vi "Process GD Infos.vi"(5 "include Timestamp":bool, 7 "show Status even if no Error":bool, 8 "Sprachliste":string[][](array[string]), 9 "GD Info-Cluster in":T1, 10 "Array (Eingang)":string[](array[string]), 11 "Error occured (Eingang)":bool) -> (1 "GD Infos":string, 2 "Array (Ausgang)":string[](array[string]), 3 "Error occured (Ausgang)":bool)   [LabVIEW 2020, in "Linearisierung v2.lvlib" / "SpanEinstellungen.lvlib"]
uses:
  SpanEinstellungen.lvlib
  GD Info Cluster.ctl
  LIN ErrorCluster.ctl
  Sprachverwaltung/Sprachverwaltung.lvlib
  Linearisierung v2.lvlib
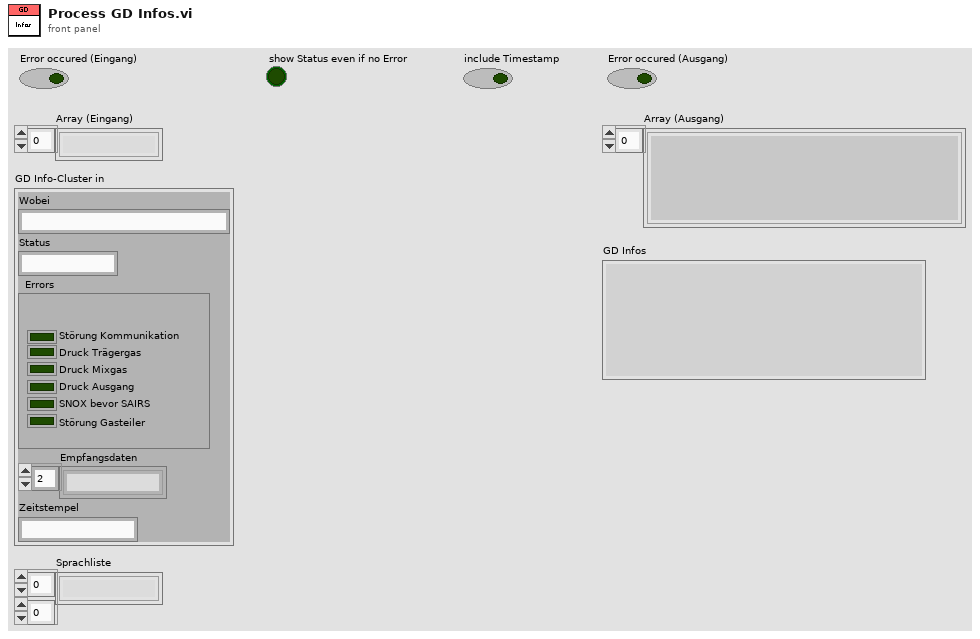
[diagram p1: front panel]
types:
  T1 = typedef "Linearisierung v2.lvlib/SpanEinstellungen.lvlib/GD Info Cluster.ctl" = cluster{"Wobei":string, "Status":string, "Errors":T2, "Empfangsdaten":string[], "Zeitstempel":string}
  T2 = typedef "Linearisierung v2.lvlib/LIN ErrorCluster.ctl" = cluster{"Störung Kommunikation":bool, "Pressure carrier gas":bool, "Pressure diluted gas":bool, "Outlet Pressure":bool, "SNOX before SAIR":bool, "Störung Gasteiler":bool}
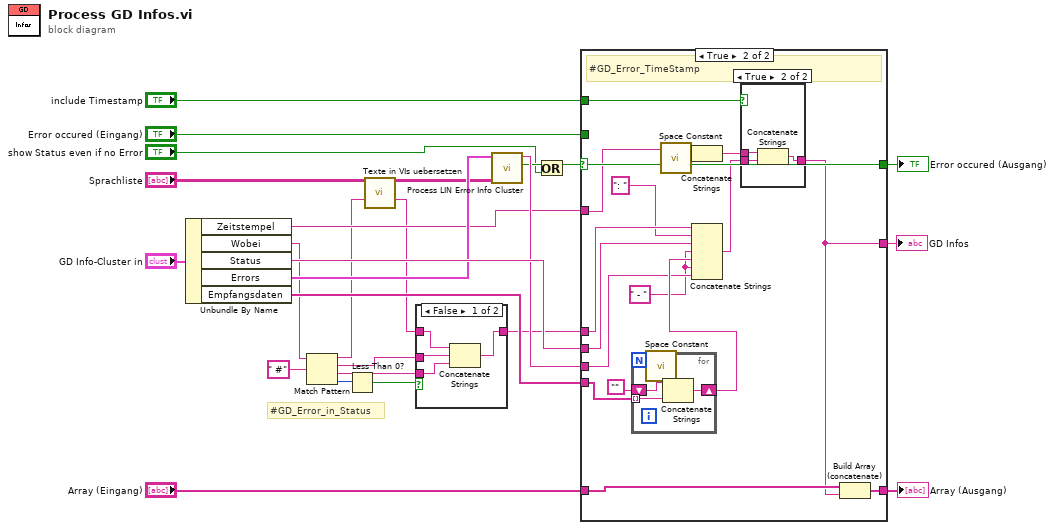
[diagram p0: block diagram]
diagram:
  # "#GD_Error_in_Status"
  n1 = Unbundle By Name("GD Info-Cluster in") -> ("Zeitstempel"=w13:string, "Wobei"=w9:string, "Status"=w21:string, "Errors"=w18:T2, "Empfangsdaten"=w22:string[])
  n2 = Match Pattern(string=w9, regular expression=" #" ("Regulärer Ausdruck")) -> (before substring=w5:string, match substring=w2:string, after substring=w1:string, offset past match=w7:i32)  [unwired: 1 in]
  n3 = Less Than 0?(x=w7) -> (x < 0?=w6:bool)
  n4 = call "Texte in VIs uebersetzen.vi"("Sprachliste"="Sprachliste", "String zum Übersetzen"=w5) -> ("Sprachliste out"=w10:string[][], "String zum Übersetzen"=w4:string)  [unwired: 9 in, 3 out]
  n5 = case shown="False" w6 {
    tunnel: w4 -> [w30 w31]
    tunnel: [w27 w31] -> w3
    tunnel: w2 -> [w29 _]
    tunnel: w1 -> [w28 _]
    frame False {
      n6 = Concatenate Strings(w30, w29, w28) -> (w27:string)
    }
    frame True {
    }
  }
  n7 = call "Process LIN Error Info Cluster.vi"("Sprachliste"=w10, "Errors"=w18) -> ("Störung"=w19:bool, "String"=w20:string)  [unwired: 8 in]
  n8 = Or(x=w19, y="show Status even if no Error") -> (x .or. y?=w15:bool)
  n9 = case shown="True" w15 {
    selector: w15 -> [_ w43]
    tunnel: w20 -> [_ w46]
    tunnel: w3 -> [_ w49]
    tunnel: w21 -> [_ w48]
    tunnel: w22 -> [_ w50]
    tunnel: [w33 w45] -> w23
    tunnel: "Array (Eingang)" -> [w33 w44]
    tunnel: [w32 w43] -> w25
    tunnel: "Error occured (Eingang)" -> [w32 _]
    tunnel: [_ w34] -> w16
    tunnel: w13 -> [_ w39]
    tunnel: "include Timestamp" -> [_ w37]
    frame False {
    }
    frame True {
      w40 = " - "
      # "#GD_Error_TimeStamp"
      n10 = for {
        tunnel: w50 -> [w58] mode=indexing
        shift-right: [w57] -> w47
        shift-left: "" -> [w56]
        n11 = call <vilib>:"Space Constant.vi"() -> ("String"=w55:string)
        n12 = Concatenate Strings(w56, w55, w58) -> (w57:string)
      }
      n13 = call <vilib>:"Space Constant.vi"() -> ("String"=w38:string)
      n14 = Concatenate Strings(w39, w38) -> (w36:string)
      n15 = Concatenate Strings(w49, ": ", w48, w40, w47, w40, w46) -> (w35:string)
      n16 = case shown="True" w37 {
        tunnel: w36 -> [_ w54]
        tunnel: w35 -> [w51 w53]
        tunnel: [w51 w52] -> w34
        frame False {
        }
        frame True {
          n17 = Concatenate Strings(w54, w53) -> (w52:string)
        }
      }
      n18 = Build Array (concatenate)(w44, w34) -> (w45:string[])
    }
  }
  "Error occured (Ausgang)" <- w25
  "Array (Ausgang)" <- w23
  "GD Infos" <- w16
